vi "XW_file_info.vi"(0 "Instrument type":T1=enum."Cross wire angle", 1 "Ch No":i16) -> (2 "Filename":path, 3 "resulting string":string, 4 "File Exists?":bool)   [LabVIEW 2020]
uses:
  Controls/Cal_Inst_type.ctl
  File/Setup_Filetype.ctl
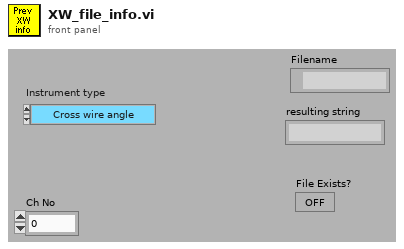
[diagram p1: front panel]
types:
  T1 = typedef "Cal_Inst_type.ctl" = enum16{"Propeller anemometer", "Pressure Transducer", "Hot wire", "Cross wire velocity", "Cross wire angle", "Generic Linear", "Generic Polynomial", "Generic BackPoly", "Fast FID", "Thermocouple", "Cold wire", "Pulsed Wire"}
  T2 = typedef "Setup_Filetype.ctl" = enum16{"Measurement Setups", "Calibration Setups", "General", "Results File Plotter Setups", "Speed Calib Tweaks"}
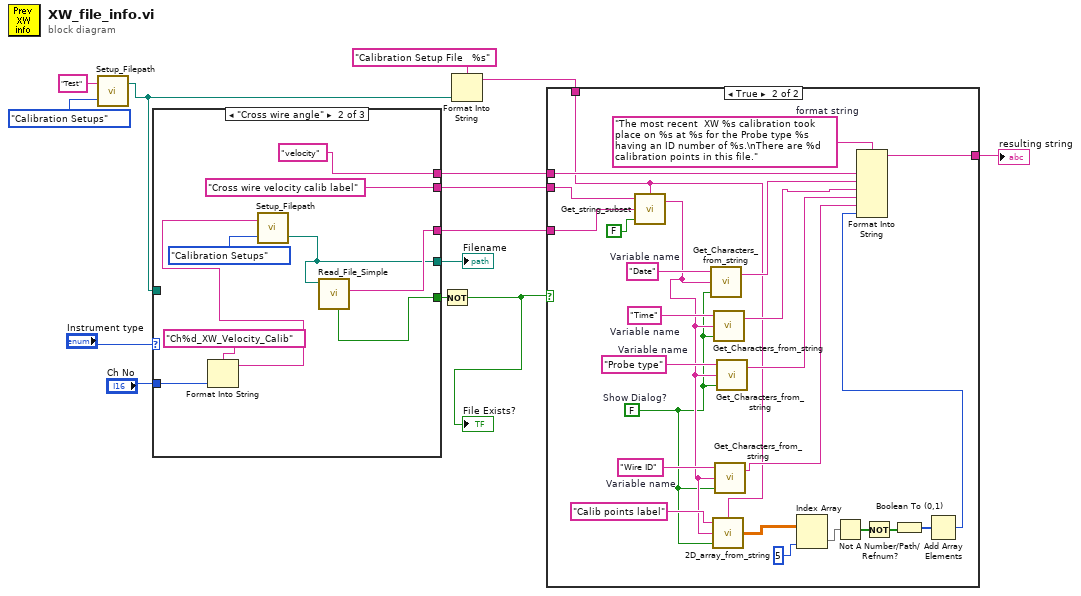
[diagram p0: block diagram]
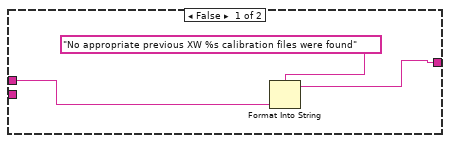
[diagram p2: hidden frame]
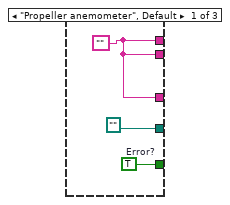
[diagram p3: hidden frame]
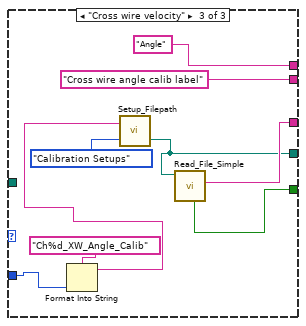
[diagram p4: hidden frame]
diagram:
  n1 = call "Setup_Filepath.vi"("Setup File Type"=Setup_Filetype."Calibration Setups", "Filename in"="Test") -> ("Directory"=w2:path)  [unwired: 1 out]
  n2 = case shown="\"Cross wire angle\"" "Instrument type" {
    tunnel: w2 -> [_ _ _]
    tunnel: [w17 w26 w35] -> w13
    tunnel: [w16 "Cross wire velocity calib label" "Cross wire angle calib label"] -> w11
    tunnel: [w16 w24 w33] -> w10
    tunnel: [w16 "velocity" "Angle"] -> w9
    tunnel: [path "" w18 w27] -> w7
    tunnel: "Ch No" -> [_ w21 w30]
    frame "Propeller anemometer", Default {
      w16 = ""
      w17 = TRUE  # Error?
    }
    frame "Cross wire angle" {
      n3 = Format Into String(format string="Ch%d_XW_Velocity_Calib", w21) -> (resulting string=w19:string)  [unwired: 2 in, 1 out]
      n4 = call "Setup_Filepath.vi"("Setup File Type"=Setup_Filetype."Calibration Setups", "Filename in"=w19) -> ("Filename Out"=w18:path)  [unwired: 1 out]
      n5 = call "Read_File_Simple.vi"("Filename"=w18) -> ("Error?"=w26:bool, "string"=w24:string)  [unwired: 2 in, 6 out]
    }
    frame "Cross wire velocity" {
      n6 = Format Into String(format string="Ch%d_XW_Angle_Calib", w30) -> (resulting string=w28:string)  [unwired: 2 in, 1 out]
      n7 = call "Setup_Filepath.vi"("Setup File Type"=Setup_Filetype."Calibration Setups", "Filename in"=w28) -> ("Filename Out"=w27:path)  [unwired: 1 out]
      n8 = call "Read_File_Simple.vi"("Filename"=w27) -> ("Error?"=w35:bool, "string"=w33:string)  [unwired: 2 in, 6 out]
    }
  }
  "Filename" <- w7
  n9 = Not(x=w13) -> (.not. x?=w12:bool)
  "File Exists?" <- w12
  n10 = Format Into String(format string="Calibration Setup File   %s", w2) -> (resulting string=w4:string)  [unwired: 2 in, 1 out]
  n11 = case shown="True" w12 {
    tunnel: w11 -> [_ w62]
    tunnel: w10 -> [_ w61]
    tunnel: w9 -> [w37 w57]
    tunnel: [w36 w54] -> w8
    tunnel: w4 -> [_ w39]
    frame False {
      n12 = Format Into String(format string="No appropriate previous XW %s calibration files were found", w37) -> (resulting string=w36:string)  [unwired: 2 in, 1 out]
    }
    frame True {
      w46 = "Time"  # Variable name
      w55 = "Wire ID"  # Variable name
      w56 = "The most recent  XW %s calibration took place on %s at %s for the Probe type %s having an ID number of %s.\nThere are %d calibration points in this file."  # format string
      w44 = FALSE  # Show Dialog?
      w59 = "Probe type"  # Variable name
      w60 = "Date"  # Variable name
      n13 = call "Get_string_subset.vi"("String Name"=w39, "Show Dialog?"=FALSE, "String to split"=w61, "File Label"=w62) -> ("Output string"=w45:string)  [unwired: 1 out]
      n14 = call "Get_Characters_from_string.vi"("Show Dialog?"=w44, "Input string"=w45, "Variable name"=w60) -> ("Value"=w58:string)  [unwired: 1 out]
      n15 = call "2D_array_from_string.vi"("String Name"=w39, "Show Dialog?"=w44, "Input string"=w45, "Array title"="Calib points label") -> ("2D data array"=w52:dbl[][])
      n16 = call "Get_Characters_from_string.vi"("Show Dialog?"=w44, "Input string"=w45, "Variable name"=w46) -> ("Value"=w43:string)  [unwired: 1 out]
      n17 = call "Get_Characters_from_string.vi"("Show Dialog?"=w44, "Input string"=w45, "Variable name"=w55) -> ("Value"=w41:string)  [unwired: 1 out]
      n18 = call "Get_Characters_from_string.vi"("Show Dialog?"=w44, "Input string"=w45, "Variable name"=w59) -> ("Value"=w42:string)  [unwired: 1 out]
      n19 = Index Array(array=w52, index (col)=5 ("Index")) -> (element=w50:dbl[])  [unwired: 1 in]
      n20 = Not A Number/Path/Refnum?(number/path/refnum=w50) -> (NaN/Path/Refnum?=w49:bool[])
      n21 = Not(x=w49) -> (.not. x?=w48:bool[])
      n22 = Boolean To (0,1)(Boolean=w48) -> (0, 1=w47:i16[])
      n23 = Add Array Elements(numeric array=w47) -> (sum=w40:i16)
      n24 = Format Into String(format string=w56, w57, w58, w43, w42, w41, w40) -> (resulting string=w54:string)  [unwired: 2 in, 1 out]
    }
  }
  "resulting string" <- w8
